vi "Configure Surge-Drop.vi"(0 "VISA resource name":refnum<visa-resource-name>, 1 "Enable Surge Drop (F:Disable)":bool, 2 "Enable  Continuous Surge Drop (F:Disable)":bool, 5 "Surge Drop Voltage (100 V)":dbl=100.0 min=0.0 max=300.0 format="%.1f", 7 "Surge Drop Start Time (0 ms)":dbl min=0.0 max=99.0, 9 "Surge Drop Duration (0 ms)":dbl min=0.0 max=99.0, 11 "error in (no error)":errorcluster) -> (4 "VISA resource name out":refnum<visa-resource-name>, 15 "error out":errorcluster)   [LabVIEW 2020, in "eec 6700.lvlib"]
doc: "Configures the Surge-Drop in the active step of the power source instrument.\n\nSurge / Drop - Associated Power Technologies feature that allows the instrument to simulate loading, brown outs or voltage dips.\n\nNote :\n1. Firmware version 2.0 :\nProgram Mode : Step Parameter (Can be configured in every step individually).\nManual Mode : System Parameter ( Change in mode affect all steps and memory)\nDC Mode : Not Supported\n\n2.Firmware version 1.06 : \nProgram Mode : System Parameter ( Change in mode affect all steps and memory)\nManual Mode : System Parameter ( Change in mode affect all steps and memory)\nDC Mode : Not Supported"
uses:
  <instrlib>/EEC6700LV-driver/eec 6700.lvlib
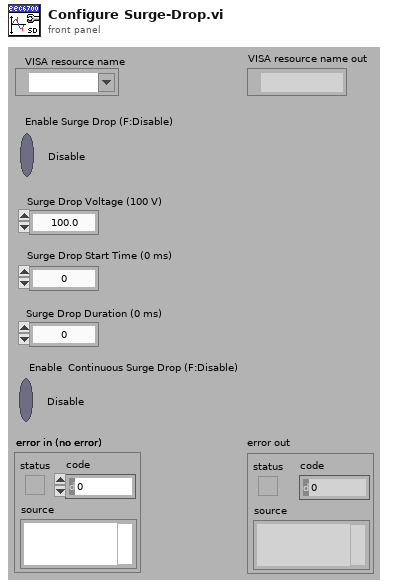
[diagram p1: front panel]
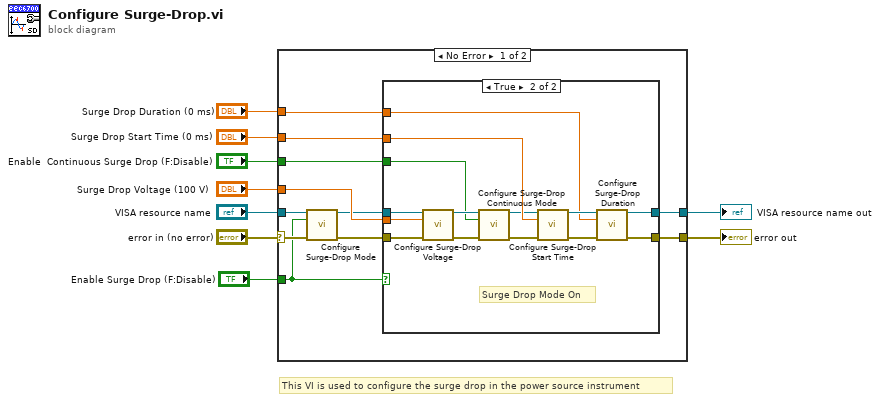
[diagram p0: block diagram]
diagram:
  # "This VI is used to configure the surge drop in the power source instrument"
  n1 = case shown="No Error" "error in (no error)" {
    selector: "error in (no error)" -> [w12 w38]
    tunnel: [w20 w38] -> w9
    tunnel: [w19 w37] -> w8
    tunnel: "VISA resource name" -> [w15 w37]
    tunnel: "Surge Drop Voltage (100 V)" -> [w18 _]
    tunnel: "Surge Drop Start Time (0 ms)" -> [w17 _]
    tunnel: "Surge Drop Duration (0 ms)" -> [w16 _]
    tunnel: "Enable  Continuous Surge Drop (F:Disable)" -> [w10 _]
    tunnel: "Enable Surge Drop (F:Disable)" -> [w11 _]
    frame No Error {
      n2 = call <instrlib>:"Configure Surge-Drop Mode.vi"("VISA resource name"=w15, "Enable Surge Drop (F:Disable)"=w11, "error in (no error)"=w12) -> ("VISA resource name out"=w14:refnum<visa-resource-name>, "error out"=w13:errorcluster)  [unwired: 11 in]
      n3 = case shown="True" w11 {
        tunnel: [w21 w28] -> w20
        tunnel: [w22 w29] -> w19
        tunnel: w18 -> [_ w34]
        tunnel: w17 -> [_ w33]
        tunnel: w16 -> [_ w32]
        tunnel: w14 -> [w22 w31]
        tunnel: w13 -> [w21 w30]
        tunnel: w10 -> [_ w23]
        frame False {
          # "Surge Drop Mode Off"
        }
        frame True {
          # "Surge Drop Mode On"
          n4 = call <instrlib>:"Configure Surge-Drop Voltage.vi"("VISA resource name"=w31, "Surge Drop Voltage (100 V)"=w34, "error in (no error)"=w30) -> ("VISA resource name out"=w27:refnum<visa-resource-name>, "error out"=w25:errorcluster)  [unwired: 11 in]
          n5 = call <instrlib>:"Configure Surge-Drop Continuous Mode.vi"("VISA resource name"=w27, "Enable  Continuous Surge Drop (F:Disable)"=w23, "error in (no error)"=w25) -> ("VISA resource name out"=w26:refnum<visa-resource-name>, "error out"=w24:errorcluster)  [unwired: 11 in]
          n6 = call <instrlib>:"Configure Surge-Drop Start Time.vi"("VISA resource name"=w26, "Surge Drop Start Time (0 ms)"=w33, "error in (no error)"=w24) -> ("VISA resource name out"=w36:refnum<visa-resource-name>, "error out"=w35:errorcluster)  [unwired: 11 in]
          n7 = call <instrlib>:"Configure Surge-Drop Duration.vi"("VISA resource name"=w36, "Surge Drop Duration (0 ms)"=w32, "error in (no error)"=w35) -> ("VISA resource name out"=w29:refnum<visa-resource-name>, "error out"=w28:errorcluster)  [unwired: 11 in]
        }
      }
    }
    frame Error {
    }
  }
  "error out" <- w9
  "VISA resource name out" <- w8
